vi "Error to Message.vi"(8 "Error In":errorcluster) -> (0 "Error Out":errorcluster, 3 "Error Message":string)   [LabVIEW 2016, in "CS++Utilities.lvlib"]
doc: "Get erro message from error in, using pure error cluster info on RT and FPGA and else Simple Error Handler."
uses:
  CS++Utilities.lvlib
  <vilib>/Utility/error.llb/DialogType.ctl
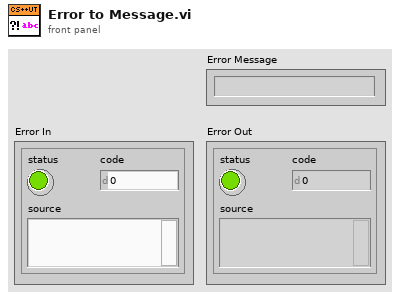
[diagram p1: front panel]
types:
  T1 = typedef "DialogType.ctl" = u16
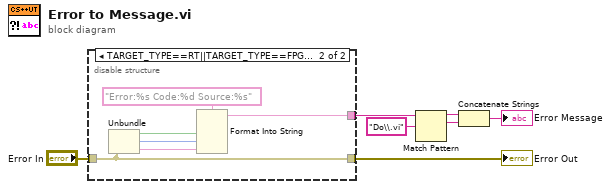
[diagram p0: block diagram]
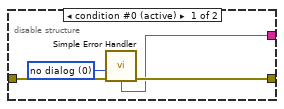
[diagram p2: hidden frame]
diagram:
  n1 = disable-structure shown="TARGET_TYPE==RT||TARGET_TYPE==FPGA" {
    disable-tunnel: "Error In" -> [w11 w16]
    disable-tunnel: [w8 w17] -> w1
    disable-tunnel: [w10 w16] -> w6
    frame condition #0 (active) {
      w9 = T1 0 items=["no dialog", "OK message", "continue or stop message", "OK message + warnings", "continue/stop + warnings"] ("type of dialog (OK msg:1)")
      n2 = call <vilib>:"Simple Error Handler.vi"("type of dialog (OK msg:1)"=w9, "error in (no error)"=w11) -> ("error out"=w10:errorcluster, "message"=w8:string)  [unwired: 3 in, 3 out]
    }
    frame condition #1 {
      n3 = Unbundle(w16) -> ("status"=w15:bool, "code"=w14:i32, "source"=w13:string)
      n4 = Format Into String(format string="Error:%s Code:%d Source:%s", w15, w14, w13) -> (resulting string=w17:string)  [unwired: 2 in, 1 out]
    }
  }
  "Error Out" <- w6
  n5 = Match Pattern(string=w1, regular expression="Do\\.vi") -> (before substring=w4:string, match substring=w3:string)  [unwired: 1 in, 2 out]
  n6 = Concatenate Strings(w4, w3) -> (→"Error Message":string)
